vi "Register for Actor Stop Event.vi"(8 "error in (no error)":errorcluster, 9 "Event Registration Refnum in":refnum<event-registration>, 11 "cRIO-CO2 in":refnum<class "cRIO-CO2.lvclass">) -> (0 "error out":errorcluster, 1 "Event Registration Refnum":refnum<event-registration>, 3 "cRIO-CO2 out":refnum<class "cRIO-CO2.lvclass">)   [LabVIEW 2015, in "cRIO-Carbondioxide.lvlib" / "cRIO-CO2.lvlib" / "cRIO-CO2.lvclass"]
uses:
  cRIO-CO2.lvclass
  cRIO-CO2.lvclass/cRIO-CO2.ctl
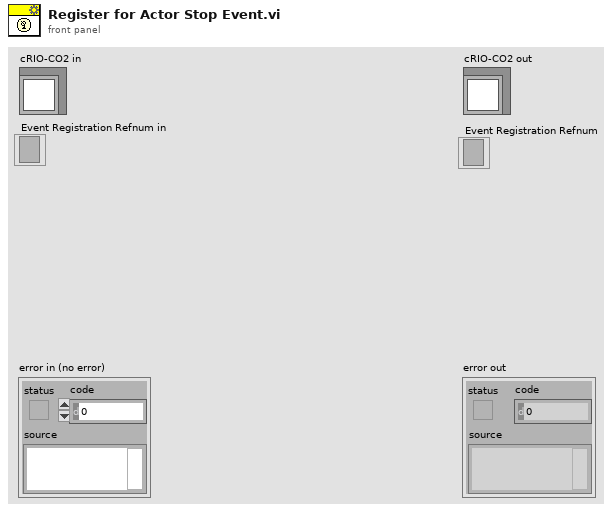
[diagram p1: front panel]
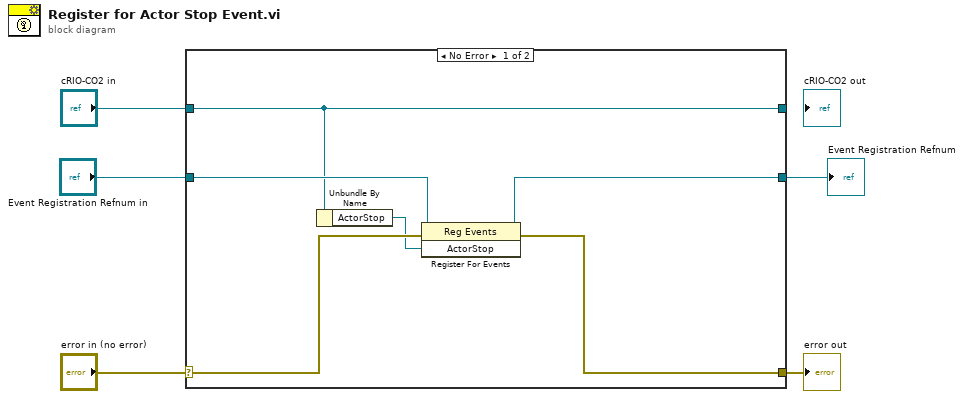
[diagram p0: block diagram]
diagram:
  n1 = case shown="No Error" "error in (no error)" {
    selector: "error in (no error)" -> [w8 w14]
    tunnel: [w9 w14] -> w4
    tunnel: [w7 w13] -> _
    tunnel: "cRIO-CO2 in" -> [w7 w13]
    tunnel: [w10 w12] -> w2
    tunnel: "Event Registration Refnum in" -> [w11 w12]
    frame No Error {
      n2 = Unbundle By Name(w7) -> ("ActorStop"=w6:refnum<user-event>)
      n3 = register-events(reference=w11, error in=w8, w6) -> (reference out=w10:refnum<event-registration>, error out=w9:errorcluster)
    }
    frame Error {
    }
  }
  "error out" <- w4
  "Event Registration Refnum" <- w2
